vi "MEMR-Find Peak.vi"(0 "Gain spectra":cluster{"Freq (Hz)":dbl[], "Mag":dbl[][]}[](array[cluster]), 7 "Mag spectra":cluster{"Freq (Hz)":dbl[], "Mag":dbl[][]}[](array[cluster]), 9 "Threshold":T1) -> (8 "Fpeak":dbl[](array[numeric]))   [LabVIEW 2020]
uses:
  MEMR-Offline Analysis Parameters.ctl
  Utility VIs/Array Manipulation VIs/Irregular Array Subset (DBL).vi
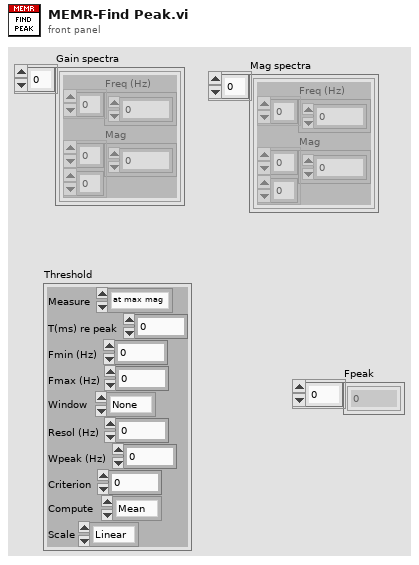
[diagram p1: front panel]
types:
  T1 = typedef "MEMR-Offline Analysis Parameters.ctl" = cluster{"Measure":enum16{"at max mag", "at max gain", "over window", "optimize", "Keefe"}, "T(ms) re peak":dbl, "Fmin (Hz)":dbl, "Fmax (Hz)":dbl, "Window":enum16{"None", "Hanning", "Hamming"}, "Resol (Hz)":dbl, "Wpeak (Hz)":dbl, "Criterion":dbl, "Compute":enum16{"Mean", "Sum"}, "Scale":enum16{"Linear", "Log"}}
  T2 = enum16{"at max mag", "at max gain", "over window"}
  T3 = enum16{"at max mag", "at max gain", "over window", "optimize", "Keefe"}
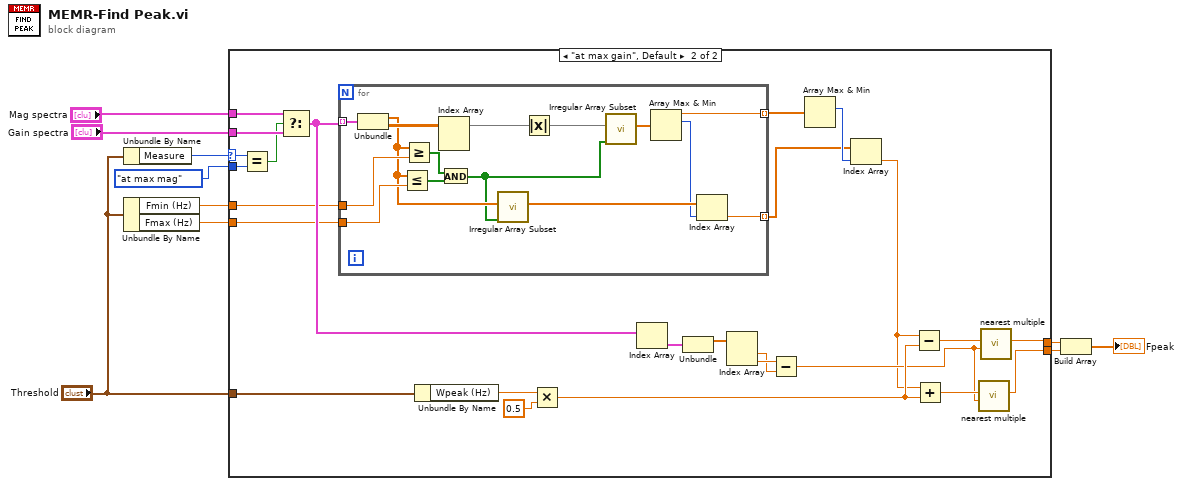
[diagram p0: block diagram]
diagram:
  n1 = Unbundle By Name("Threshold") -> ("Measure"=w7:T3)
  n2 = Unbundle By Name("Threshold") -> ("Fmin (Hz)"=w3:dbl, "Fmax (Hz)"=w2:dbl)
  n3 = case shown="\"at max gain\", Default" w7 {
    selector: w7 -> [_ w23]
    tunnel: [w12 w25] -> w10
    tunnel: [w11 w24] -> w9
    tunnel: "Mag spectra" -> [_ w22]
    tunnel: "Gain spectra" -> [_ w21]
    tunnel: "Threshold" -> [_ w18]
    tunnel: w3 -> [w12 w17]
    tunnel: w2 -> [w11 w16]
    tunnel: T2."at max mag" ("y") -> [_ w13]
    frame "over window" {
    }
    frame "at max gain", Default {
      n4 = Equal?(x=w23, y=w13) -> (x = y?=w20:bool)
      n5 = Select(t=w22, s=w20, f=w21) -> (s? t:f=w19:cluster{"Freq (Hz)":dbl[], "Mag":dbl[][]}[])
      n6 = for {
        tunnel: w19 -> [w52] mode=indexing
        tunnel: [w50] -> w37 mode=indexing
        tunnel: w17 -> [w48]
        tunnel: w16 -> [w45]
        tunnel: [w41] -> w15 mode=indexing
        n7 = Unbundle(w52) -> ("Freq (Hz)"=w44:dbl[], "Mag"=w51:dbl[][])
        n8 = Less Or Equal?(x=w44, y=w45) -> (x <= y?=w47:bool[])
        n9 = Greater Or Equal?(x=w44, y=w48) -> (x >= y?=w46:bool[])
        n10 = Index Array(array=w51) -> (element=w40:dbl[])  [unwired: 2 in]
        n11 = And(x=w46, y=w47) -> (x .and. y?=w43:bool[])
        n12 = call-poly "Irregular Array Subset.vi"("Mask"=w43, "Array"=w44) -> ("Array Subset"=w42:dbl[])  [unwired: 8 in, 1 out]
        n13 = Absolute Value(x=w40) -> (abs(x)=w49:dbl[])
        n14 = call-poly "Irregular Array Subset.vi"("Mask"=w43, "Array"=w49) -> ("Array Subset"=w39:dbl[])  [unwired: 8 in, 1 out]
        n15 = Array Max & Min(array=w39) -> (max value=w50:dbl, max index (indices)=w38:i32)  [unwired: 2 out]
        n16 = Index Array(array=w42, index=w38) -> (element=w41:dbl)
      }
      n17 = Unbundle By Name(w18) -> ("Wpeak (Hz)"=w34:dbl)
      n18 = Multiply(x=w34, y=0.5) -> (x*y=w28:dbl)
      n19 = Index Array(array=w19) -> (element=w35:cluster{"Freq (Hz)":dbl[], "Mag":dbl[][]})  [unwired: 1 in]
      n20 = Unbundle(w35) -> ("Freq (Hz)"=w32:dbl[])  [unwired: 1 out]
      n21 = Index Array(array=w32) -> (element #1=w30:dbl, element #2=w31:dbl)  [unwired: 2 in]
      n22 = Subtract(x=w31, y=w30) -> (x-y=w26:dbl)
      n23 = Array Max & Min(array=w37) -> (max index (indices)=w36:i32)  [unwired: 3 out]
      n24 = Index Array(array=w15, index=w36) -> (element=w14:dbl)
      n25 = Subtract(x=w14, y=w28) -> (x-y=w29:dbl)
      n26 = Add(x=w14, y=w28) -> (x+y=w27:dbl)
      n27 = call "nearest multiple.vi"("y"=w26, "x"=w27) -> ("round(x/y)*y"=w24:dbl)  [unwired: 7 in, 2 out]
      n28 = call "nearest multiple.vi"("y"=w26, "x"=w29) -> ("round(x/y)*y"=w25:dbl)  [unwired: 7 in, 2 out]
    }
  }
  n29 = Build Array(w10, w9) -> (→"Fpeak":dbl[])
